vi "TBA_NET_Symbol To Image.vi"(8 "Error In":errorcluster caption="错误输入（无错误）", 11 "IconPath":path) -> (0 "Error Out":errorcluster caption="错误输入（无错误）", 3 "Image":refnum<k24>)   [LabVIEW 2016]
uses:
  System.Drawing
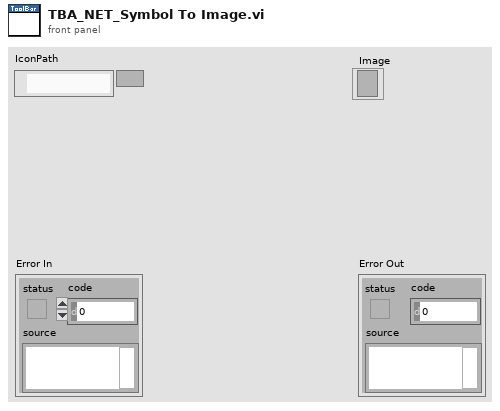
[diagram p1: front panel]
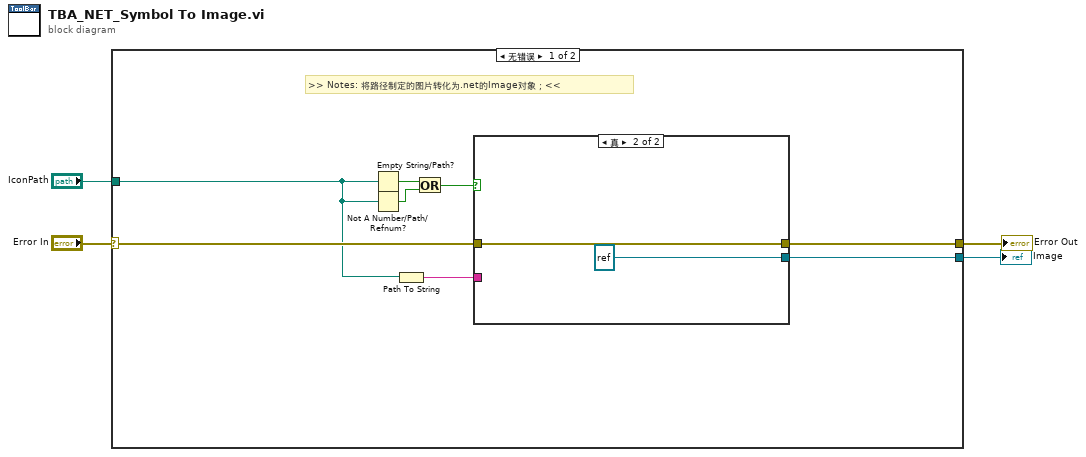
[diagram p0: block diagram]
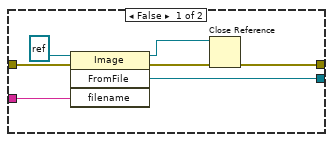
[diagram p2: hidden frame]
diagram:
  n1 = case shown="无错误" "Error In" {
    selector: "Error In" -> [w7 w22]
    tunnel: [w8 w22] -> w3
    tunnel: [w6 _] -> w2
    tunnel: "IconPath" -> [w5 _]
    frame No Error {
      # ">> Notes: 将路径制定的图片转化为.net的Image对象；<<"
      n2 = Empty String/Path?(string/path=w5) -> (empty?=w11:bool)
      n3 = Not A Number/Path/Refnum?(number/path/refnum=w5) -> (NaN/Path/Refnum?=w10:bool)
      n4 = Path To String(path=w5) -> (string=w12:string)
      n5 = Or(x=w11, y=w10) -> (x .or. y?=w9:bool)
      n6 = case shown="真" w9 {
        tunnel: w12 -> [w19 _]
        tunnel: [w18 refnum<k24> refnum ("FromFile")] -> w6
        tunnel: w7 -> [w17 w21]
        tunnel: [w13 w21] -> w8
        frame False {
          n7 = invoke class="Image" method="FromFile"(reference=refnum<k24> refnum ("引用"), error in=w17, "filename"=w19) -> (reference out=w15:refnum<k24>, error out=w14:errorcluster, "FromFile"=w18:refnum<k24>)  [unwired: 1 in, 1 out]
          n8 = Close Reference(reference=w15, error in (no error)=w14) -> (error out=w13:errorcluster)
        }
        frame True {
        }
      }
    }
    frame Error {
    }
  }
  "Error Out" <- w3
  "Image" <- w2
